vi "stdin.write.vi"(8 "error in (no error)":errorcluster, 10 "stdin":string, 11 "dotnet_system_exec in":refnum<class "dotnet_system_exec.lvclass">) -> (0 "error out":errorcluster, 3 "dotnet_system_exec out":refnum<class "dotnet_system_exec.lvclass">)   [LabVIEW 2013, in "dotnet_system_exec.lvclass"]
doc: "Sends a line to the .NET process via stdin. This vi accepts multiline inputs in case multiple lines want to be sent at once."
uses:
  dotnet_system_exec.lvclass
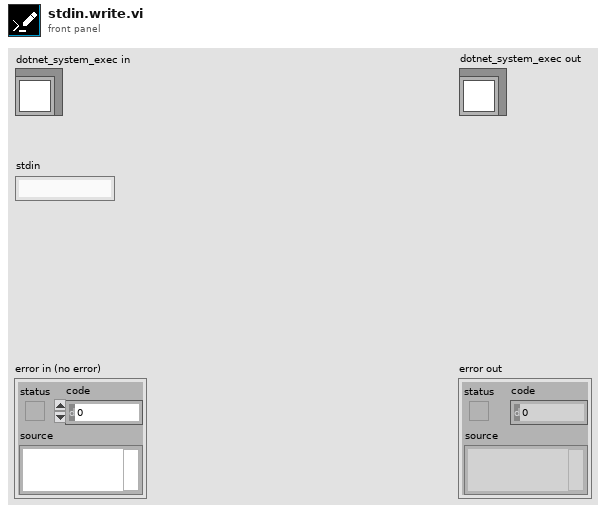
[diagram p1: front panel]
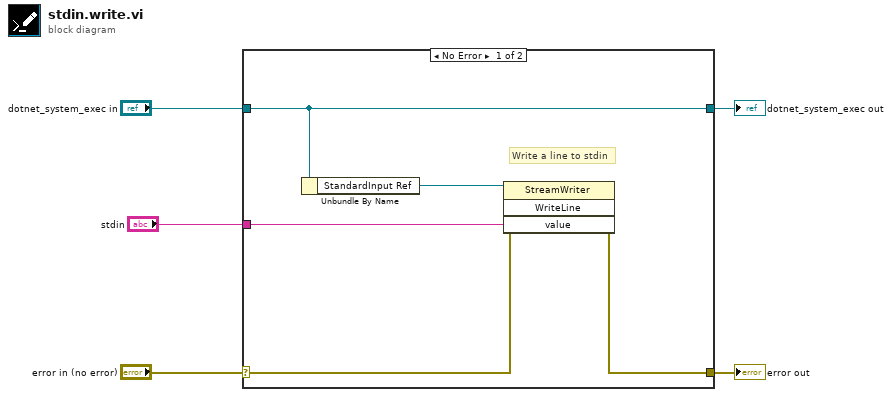
[diagram p0: block diagram]
diagram:
  n1 = case shown="No Error" "error in (no error)" {
    selector: "error in (no error)" -> [w8 w12]
    tunnel: [w7 w12] -> w4
    tunnel: [w10 w11] -> w2
    tunnel: "dotnet_system_exec in" -> [w10 w11]
    tunnel: "stdin" -> [w6 _]
    frame No Error {
      # "Write a line to stdin"
      n2 = Unbundle By Name(w10) -> ("StandardInput Ref"=w9:refnum<k24>)
      n3 = invoke class="StreamWriter" method="WriteLine"(reference=w9, error in=w8, "value"=w6) -> (error out=w7:errorcluster)  [unwired: 1 in, 3 out]
    }
    frame Error {
    }
  }
  "error out" <- w4
  "dotnet_system_exec out" <- w2
